vi "parseInclinationResponse.vi"(8 "error in (no error)":errorcluster, 10 "DynamicFrameParser":refnum<class "DynamicFrameParser.lvclass">, 11 "MIILC in":refnum<class "MIILC.lvclass">) -> (0 "error out":errorcluster, 3 "MIILC out":refnum<class "MIILC.lvclass">)   [LabVIEW 2016, in "RTMIILC.lvlib" / "MIILC.lvclass"]
uses:
  MIILC.lvclass
  Common_RT_Modbus/DynamicFrameParser/DynamicFrameParser.lvclass
  Common_RT_Modbus/DataTypes/ExceptionCodes.ctl
  MIILC.lvclass/MIILC.ctl
  Common_RT_Modbus/RTModbus.lvlib
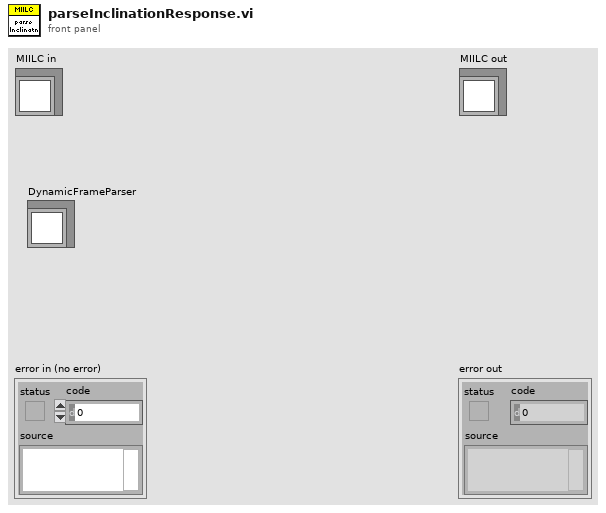
[diagram p1: front panel]
types:
  T1 = typedef "RTModbus.lvlib/ExceptionCodes.ctl" = u16
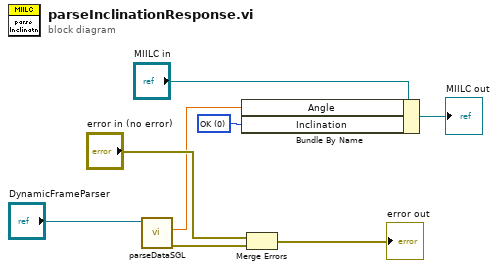
[diagram p0: block diagram]
diagram:
  w1 = T1 0 items=["OK", "IllegalFunction", "IllegalDataAddress", "IllegalDataValue", "SlaveDeviceFailure", "Acknowledge", "SlaveDeviceBusy", "NegativeAcknowledge", "MemoryParityError", "GatewayPathUnavailable", "GatewayTargetDeviceFailedToRespond"] ("MTData.MTResponses.Temperature")
  n1 = call "parseDataSGL.vi"("FrameParser in"="DynamicFrameParser") -> ("error out"=w3:errorcluster, "Data"=w5:sgl)  [unwired: 8 in, 1 out]
  n2 = Bundle By Name(cluster="MIILC in", "Angle"=w5, "Inclination"=w1) -> (→"MIILC out":refnum<class "MIILC.lvclass">)
  n3 = Merge Errors("error in (no error)", w3) -> (→"error out":errorcluster)
